vi "Image Acquirer.vi"() -> ()   [LabVIEW 2018]
uses:
  <vilib>/vision/driver/IMAQdx.llb/IMAQdx Camera Control Mode.ctl
  <vilib>/userdefined/High Color/IMAQdx.ctl
  <vilib>/vision/driver/NI_Vision_Acquisition_Software.lvlib
  <resource>/objmgr/imaqdx.rc
panel:
  in  "stop":bool
  in  "error in 3":errorcluster
  out "Image Out":T1(plugin-control)
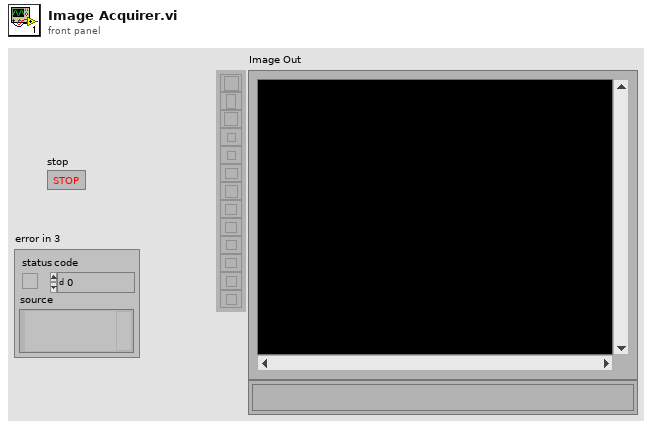
[diagram p1: front panel]
types:
  T1 = typedef "IMAQ Image.ctl" = refnum<image>
  T2 = typedef "IMAQdx.ctl" = refnum<k21>
  T3 = typedef "NI_Vision_Acquisition_Software.lvlib/IMAQdx Camera Control Mode.ctl" = enum32{"Controller", "Listener"}
  T4 = typedef "Image Type" = u32
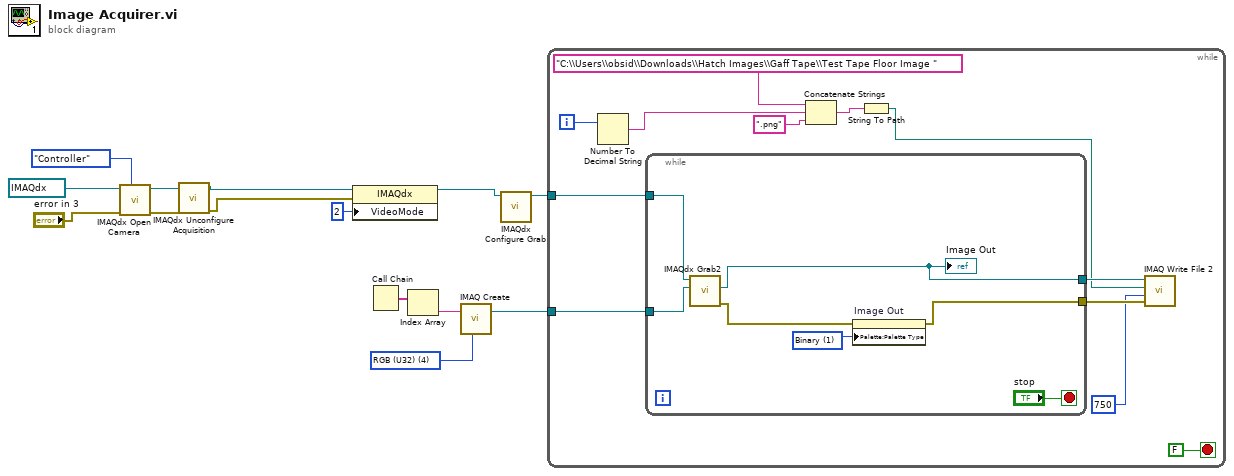
[diagram p0: block diagram]
diagram:
  w6 = T4 4 items=["Grayscale (U8)", "Grayscale (I16)", "Grayscale (SGL)", "Complex (CSG)", "RGB (U32)", "HSL (U32)", "RGB (U64)", "Grayscale (U16)"] ("Image Type")
  n1 = call <vilib>:"IMAQdx Open Camera.vi"("Camera Control Mode"=IMAQdx_Camera_Control_Mode."Controller", "error in"="error in 3", "Session In"=T2 "cam1") -> ("error out"=w11:errorcluster, "Session Out"=w12:T2)  [unwired: 7 in]
  n2 = call <vilib>:"IMAQdx Unconfigure Acquisition.vi"("error in"=w11, "Session In"=w12) -> ("error out"=w14:errorcluster, "Session Out"=w13:T2)  [unwired: 8 in]
  n3 = property class="IMAQdx"(reference=w13, error in=w14, "VideoMode"=u32 2) -> (reference out=w10:T2)  [unwired: 1 out]
  n4 = Call Chain() -> (call chain=w8:string[])
  n5 = Index Array(array=w8) -> (element=w7:string)  [unwired: 1 in]
  n6 = call "IMAQ Create"("Image Name"=w7, "Image Type"=w6) -> ("New Image"=w1:T1)  [unwired: 2 in, 2 out]
  n7 = call <vilib>:"IMAQdx Configure Grab.vi"("Session In"=w10) -> ("Session Out"=w2:T2)  [unwired: 9 in, 1 out]
  n8 = while {
    tunnel: w2 -> [w26]
    tunnel: w1 -> [w25]
    i -> [w19]
    stop <- FALSE stop-if-true
    n9 = Number To Decimal String(number=w19) -> (decimal integer string=w18:string)  [unwired: 1 in]
    n10 = while {
      tunnel: w26 -> [w32]
      tunnel: w25 -> [w31]
      tunnel: [w28] -> w24
      tunnel: [w27] -> w23
      stop <- "stop" stop-if-true
      w33 = u32 1 items=["Grayscale", "Binary", "Gradient", "Rainbow", "Temperature", "User Defined", "Binary 16 Bit", "Gradient 16 Bit", "Rainbow 16 Bit", "Temperature 16 Bit", "User Defined 16 Bit"] ("Palette Type")
      n11 = call <vilib>:"IMAQdx Grab2.vi"("Image In"=w31, "Session In"=w32) -> ("error out"=w30:errorcluster, "Image Out"=w28:T1)  [unwired: 6 in, 2 out]
      "Image Out" <- w28
      n12 = property on="Image Out" class="ImageControl"(error in=w30, "Palette:Palette Type"=w33) -> (error out=w27:errorcluster)  [unwired: 1 in, 1 out]
    }
    n13 = Concatenate Strings("C:\\Users\\obsid\\Downloads\\Hatch Images\\Gaff Tape\\Test Tape Floor Image ", w18, ".png") -> (w17:string)
    n14 = String To Path(string=w17) -> (path=w20:path)
    n15 = call-poly "IMAQ Write File 2"("error in (no error)"=w23, "Image Quality"=u32 750, "File Path"=w20, "Image"=w24) -> ()  [unwired: 6 in, 2 out]
  }
